vi "AddHeaderParams(STR).vi"(0 "gfits refnum":T1, 11 "Error in":errorcluster, 13 "IntegerLine":T2(array[cluster])) -> (4 "dup gfits refnum":T1, 15 "Error out":errorcluster)   [LabVIEW 2019]
uses:
  gfitsio/gfitsio-refnum.ctl
  gfitsio/gfitsio.lvlib
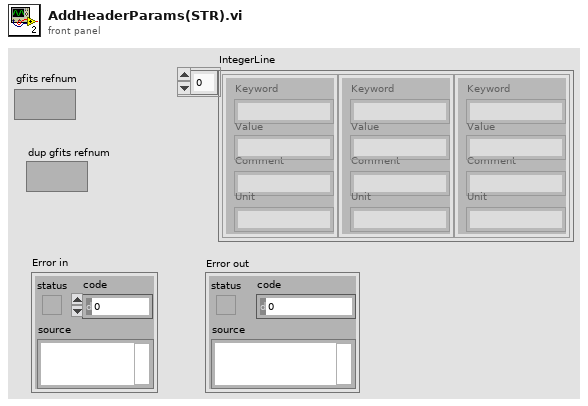
[diagram p1: front panel]
types:
  T1 = typedef "gfitsio.lvlib/gfitsio-refnum.ctl" = refnum<k1>
  T2 = cluster{"Keyword":string, "Value":string, "Comment":string, "Unit":string}[]
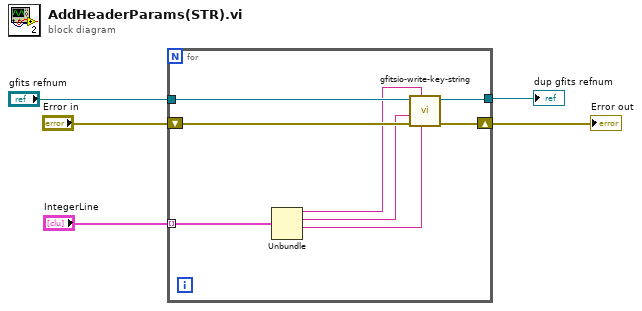
[diagram p0: block diagram]
diagram:
  n1 = for {
    tunnel: "gfits refnum" -> [w13]
    shift-right: [w11] -> w1
    shift-left: "Error in" -> [w12]
    tunnel: [w10] -> w2
    tunnel: "IntegerLine" -> [w9] mode=indexing
    n2 = Unbundle(w9) -> ("Keyword"=w8:string, "Value"=w6:string, "Comment"=w7:string)  [unwired: 1 out]
    n3 = call "gfitsio-write-key-string.vi"("comment"=w7, "keyname"=w8, "error in (no error)"=w12, "value"=w6, "gfits refnum"=w13) -> ("error out"=w11:errorcluster, "dup gfits refnum"=w10:T1)  [unwired: 5 in]
  }
  "dup gfits refnum" <- w2
  "Error out" <- w1
